vi "Add Node.vi"(8 "error in (no error)":errorcluster, 9 "Usage":string, 10 "Name":string, 11 "Tree in":refnum<class "Tree.lvclass">) -> (0 "error out":errorcluster, 2 "Node out":refnum<class "TreeNode.lvclass">, 3 "Tree out":refnum<class "Tree.lvclass">)   [LabVIEW 2013, in "MDSplus.lvlib" / "Tree.lvclass"]
doc: "Add a new node to the tree open for edit."
uses:
  <vilib>/MDSplus/Classes/Tree_Class/Tree.lvclass
  <vilib>/MDSplus/Classes/Data_Class/TreeNode_Class/TreeNode.lvclass
  <vilib>/MDSplus/Classes/Data_Class/Data.lvclass
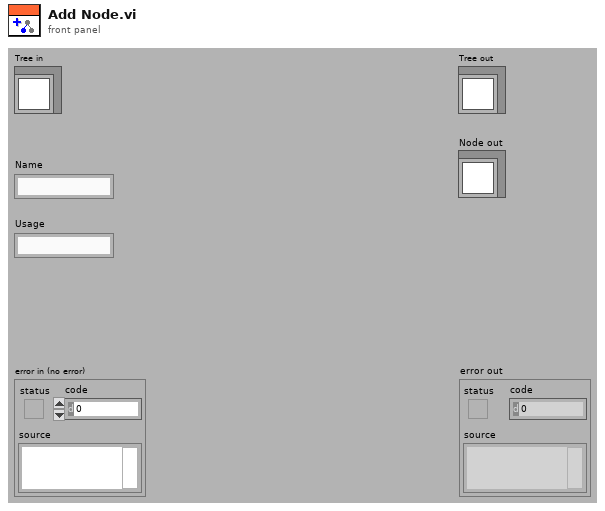
[diagram p1: front panel]
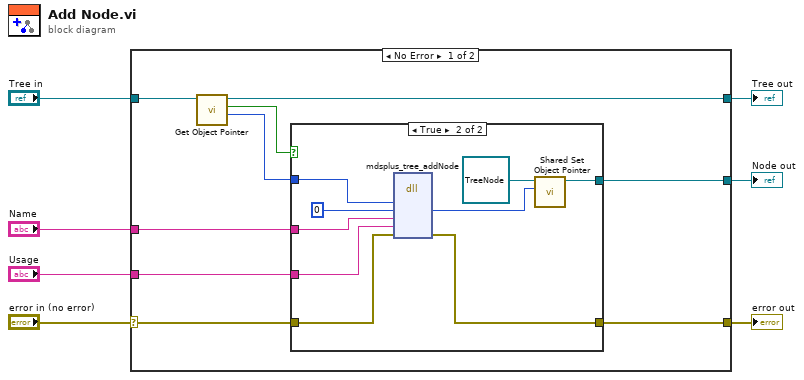
[diagram p0: block diagram]
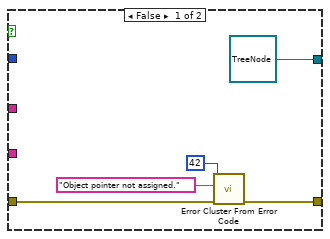
[diagram p2: hidden frame]
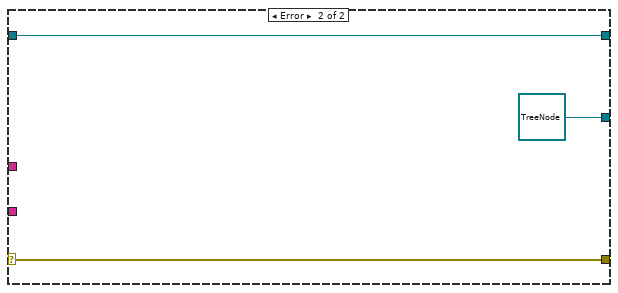
[diagram p3: hidden frame]
diagram:
  n1 = case shown="No Error" "error in (no error)" {
    selector: "error in (no error)" -> [w9 w33]
    tunnel: [w8 w33] -> w6
    tunnel: [w15 w32] -> w4
    tunnel: "Tree in" -> [w16 w32]
    tunnel: "Name" -> [w14 _]
    tunnel: "Usage" -> [w13 _]
    tunnel: [w12 refnum<class "TreeNode.lvclass"> refnum ("TreeNode out")] -> w1
    frame No Error {
      n2 = call-dynamic "Get Object Pointer.vi"("Tree in"=w16) -> ("Object Pointer"=w10:i64, "Assigned object pointer?"=w11:bool, "Tree out"=w15:refnum<class "Tree.lvclass">)  [unwired: 8 in]
      n3 = case shown="True" w11 {
        tunnel: w14 -> [_ w29]
        tunnel: w13 -> [_ w28]
        tunnel: [refnum<class "TreeNode.lvclass"> refnum ("Data out") w25] -> w12
        tunnel: w10 -> [_ w24]
        tunnel: w9 -> [w18 w23]
        tunnel: [w17 w22] -> w8
        frame False {
          n4 = call <vilib>:"Error Cluster From Error Code.vi"("error in (no error)"=w18, "error message (\"\")"="Object pointer not assigned." ("error message (\"\")"), "error code (0)"=42) -> ("error out"=w17:errorcluster)  [unwired: 6 in]
        }
        frame True {
          n5 = dll-call lib="MDSobjectsLVShr" fn="mdsplus_tree_addNode"("lvTreePtr"=w24, "lvTreeNodePtrOut"=i64 0 ("lvTreeNodePtr"), "nameIn"=w29, "usageIn"=w28, "error"=w23) -> ("lvTreeNodePtrOut"=w26:i64, "error"=w22:errorcluster)  [unwired: 7 in, 2 out]
          n6 = call <vilib>:"Shared Set Object Pointer.vi"("Object Pointer"=w26, "Data in"=refnum<class "TreeNode.lvclass"> refnum ("TreeNode")) -> ("Data out"=w25:refnum<class "TreeNode.lvclass">)  [unwired: 9 in]
        }
      }
    }
    frame Error {
    }
  }
  "error out" <- w6
  "Tree out" <- w4
  "Node out" <- w1
